vi "ASI Get ID.vi"(10 "pID":T1, 11 "iCameraID":i32) -> (2 "pID out":T1, 3 "function return":i32)   [LabVIEW 2012, in "ASICamera2_no_err.lvlib"]
doc: "ASICAMERA_API ASI_ERROR_CODE ASIGetID(int iCameraID, ASI_ID* pID);"
uses:
  <userlib>/ASICamera2_no_err/ASICamera2_no_err.lvlib
  ASICamera2.dll
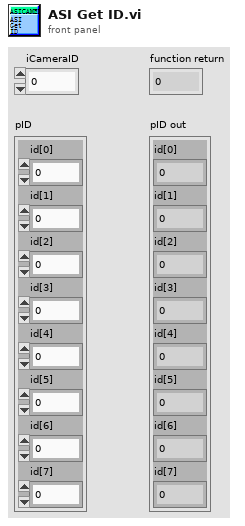
[diagram p1: front panel]
types:
  T1 = cluster{"id[0]":u8, "id[1]":u8, "id[2]":u8, "id[3]":u8, "id[4]":u8, "id[5]":u8, "id[6]":u8, "id[7]":u8}
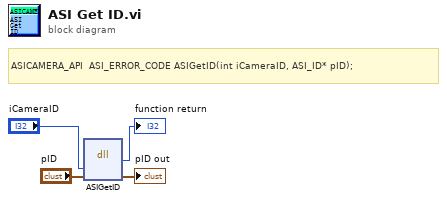
[diagram p0: block diagram]
diagram:
  # "ASICAMERA_API  ASI_ERROR_CODE ASIGetID(int iCameraID, ASI_ID* pID);"
  n1 = dll-call lib="ASICamera2.*" fn="ASIGetID"("iCameraID"="iCameraID", "pID"="pID") -> (→"function return":i32, "pID"=→"pID out":T1)  [unwired: 4 in, 2 out]
